vi "generateSignedIntegers.vi"(6 "timeout (10000)":i32=10000, 8 "error in (no error)":errorcluster, 11 "Parameters":T2={"params"={"apiKey"="", "n"=0, "min"=0, "max"=0, "replacement"=TRUE, "base"=10}, "id"=0.0} {"params"."base" items=["2"=2, "8"=8, "10"=10, "16"=16]}) -> (0 "error out":errorcluster, 3 "Response":T1={"result"={"random"={"method"="", "hashedApiKey"="", "n"=0, "min"=0, "max"=0, "replacement"=TRUE, "base"=10, "data"=[], "completionTime"="", "serialNumber"=0}, "signature"="", "bitsUsed"=0, "bitsLeft"=0, "requestsLeft"=0, "advisoryDelay"=0}, "id"=0.0} {"result"."random"."base" items=["2"=2, "8"=8, "10"=10, "16"=16]}, 4 "error data":string[](array[string]))   [LabVIEW 2014, in "Random JSON API.lvlib"]
uses:
  Random JSON API.lvlib
  Type Defs/generateIntegersRequest.ctl
  Type Defs/generateSignedIntegersResponse.ctl
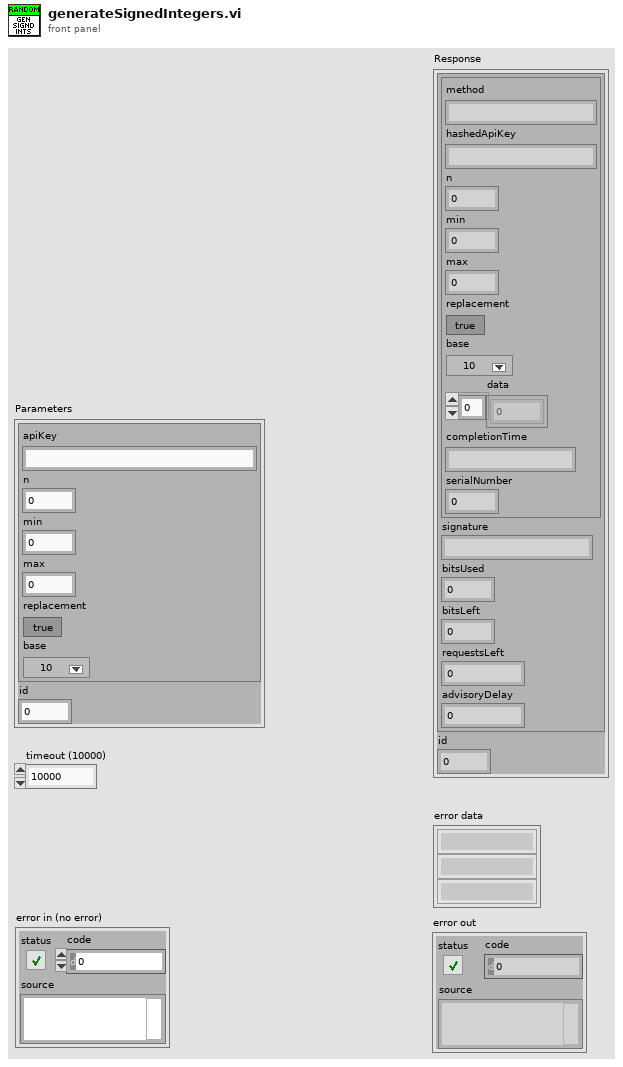
[diagram p1: front panel]
types:
  T1 = typedef "Random JSON API.lvlib/generateSignedIntegersResponse.ctl" = cluster{"result":cluster{"random":cluster{"method":string, "hashedApiKey":string, "n":i32, "min":i32, "max":i32, "replacement":bool, "base":i32, "data":i32[], "completionTime":string, "serialNumber":i32}, "signature":string, "bitsUsed":i32, "bitsLeft":i32, "requestsLeft":i32, "advisoryDelay":i32}, "id":dbl}
  T2 = typedef "Random JSON API.lvlib/generateIntegersRequest.ctl" = cluster{"params":cluster{"apiKey":string, "n":i32, "min":i32, "max":i32, "replacement":bool, "base":i32}, "id":dbl}
  T3 = cluster{"apiKey":string, "n":i32, "min":i32, "max":i32, "replacement":bool, "base":i32}
  T4 = cluster{"jsonrpc":string, "method":string, "params":cluster{"apiKey":string, "n":i32, "min":i32, "max":i32, "replacement":bool, "base":i32}, "id":dbl}
  T5 = cluster{"result cluster":cluster{"completionTime":string, "bitsUsed":i32, "bitsLeft":i32, "requestsLeft":i32, "advisoryDelay":i32}, "method":string, "hashedApiKey":string, "n":i32, "serialNumber":i32, "signature":string}
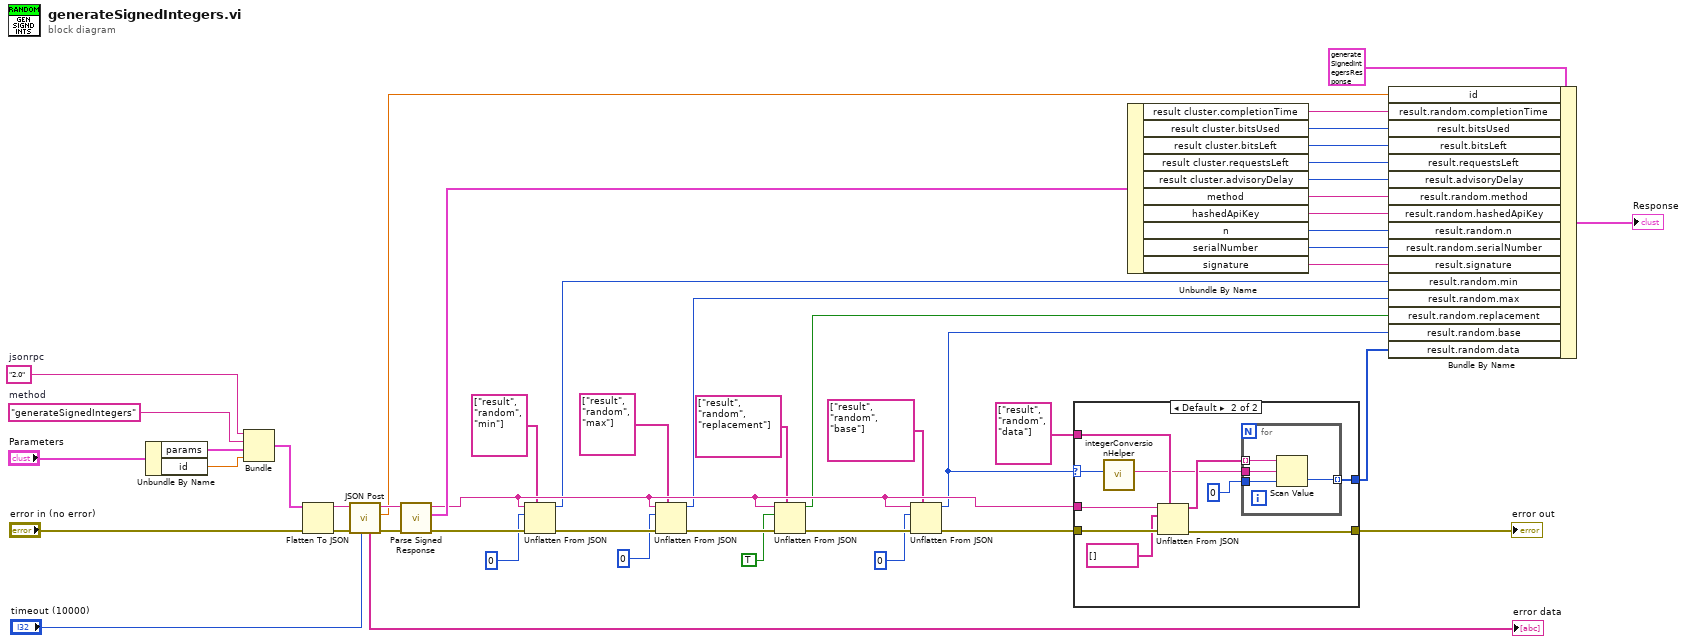
[diagram p0: block diagram]
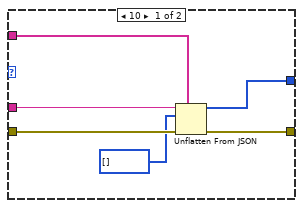
[diagram p2: hidden frame]
diagram:
  w44 = "generateSignedIntegers"  # method
  w45 = "2.0"  # jsonrpc
  n1 = Unbundle By Name("Parameters") -> ("params"=w38:T3, "id"=w37:dbl)
  n2 = Bundle("jsonrpc"=w45, "method"=w44, "params"=w38, "id"=w37) -> (w43:T4)  [unwired: 1 in]
  n3 = Flatten To JSON(anything=w43, error in (no error)="error in (no error)") -> (JSON string=w39:string, 11:w40:errorcluster)  [unwired: 1 in]
  n4 = call "JSON Post.vi"("timeout (10000)"="timeout (10000)", "error in (no error)"=w40, "Request JSON String"=w39) -> ("error out"=w47:errorcluster, "id"=w35:dbl, "Response JSON String"=w36:string, "error data"=→"error data":string[])  [unwired: 5 in]
  n5 = call "Parse Signed Response.vi"("error in (no error)"=w47, "body in"=w36) -> ("error out"=w18:errorcluster, "signed result cluster"=w34:T5, "body out"=w13:string)  [unwired: 7 in]
  n6 = Unflatten From JSON(path=string[] ["result", "random", "min"], JSON string=w13, type and defaults=0, error in (no error)=w18) -> (value=w8:i32, error out=w17:errorcluster)  [unwired: 3 in]
  n7 = Unflatten From JSON(path=string[] ["result", "random", "max"], JSON string=w13, type and defaults=0, error in (no error)=w17) -> (value=w7:i32, error out=w16:errorcluster)  [unwired: 3 in]
  n8 = Unflatten From JSON(path=string[] ["result", "random", "replacement"], JSON string=w13, type and defaults=TRUE, error in (no error)=w16) -> (value=w6:bool, error out=w15:errorcluster)  [unwired: 3 in]
  n9 = Unflatten From JSON(path=string[] ["result", "random", "base"], JSON string=w13, type and defaults=0, error in (no error)=w15) -> (value=w1:i32, error out=w14:errorcluster)  [unwired: 3 in]
  n10 = case shown="Default" w1 {
    selector: w1 -> [_ w57]
    tunnel: w14 -> [w54 w63]
    tunnel: [w53 w55] -> w46
    tunnel: [w51 w64] -> w24
    tunnel: w13 -> [w52 w61]
    tunnel: string[] ["result", "random", "data"] ("path") -> [w49 w58]
    frame 10 {
      n11 = Unflatten From JSON(path=w49, JSON string=w52, type and defaults=i32[] [], error in (no error)=w54) -> (value=w51:i32[], error out=w53:errorcluster)  [unwired: 3 in]
    }
    frame Default {
      n12 = call "integerConversionHelper.vi"("base"=w57) -> ("base conversion string"=w56:string)  [unwired: 10 in]
      n13 = Unflatten From JSON(path=w58, JSON string=w61, type and defaults=string[] [], error in (no error)=w63) -> (value=w60:string[], error out=w55:errorcluster)  [unwired: 3 in]
      n14 = for {
        tunnel: [w68] -> w64 mode=indexing
        tunnel: w60 -> [w67] mode=indexing
        tunnel: w56 -> [w65]
        tunnel: 0 -> [w66]
        n15 = Scan Value(string=w67, format string=w65, default (0 dbl)=w66) -> (value=w68:i32)  [unwired: 1 out]
      }
    }
  }
  "error out" <- w46
  n16 = Unbundle By Name(w34) -> ("result cluster.completionTime"=w33:string, "result cluster.bitsUsed"=w32:i32, "result cluster.bitsLeft"=w31:i32, "result cluster.requestsLeft"=w30:i32, "result cluster.advisoryDelay"=w29:i32, "method"=w23:string, "hashedApiKey"=w22:string, "n"=w21:i32, "serialNumber"=w20:i32, "signature"=w19:string)
  n17 = Bundle By Name(cluster=T1 {"result"={"random"={"method"="", "hashedApiKey"="", "n"=0, "min"=0, "max"=0, "replacement"=TRUE, "base"=10, "data"=[], "completionTime"="", "serialNumber"=0}, "signature"="", "bitsUsed"=0, "bitsLeft"=0, "requestsLeft"=0, "advisoryDelay"=0}, "id"=0.0} ("Response"), "id"=w35, "result.random.completionTime"=w33, "result.bitsUsed"=w32, "result.bitsLeft"=w31, "result.requestsLeft"=w30, "result.advisoryDelay"=w29, "result.random.method"=w23, "result.random.hashedApiKey"=w22, "result.random.n"=w21, "result.random.serialNumber"=w20, "result.signature"=w19, "result.random.min"=w8, "result.random.max"=w7, "result.random.replacement"=w6, "result.random.base"=w1, "result.random.data"=w24) -> (→"Response":T1)
